vi "FP_Size Inside Bounds with Scrollbars.vi"(7 "WkSpace":T1, 8 "Error":errorcluster, 11 "VI":refnum<vi>) -> (0 "Error Out":errorcluster, 2 "Fit Successful":bool, 3 "VI Out":refnum<vi>)   [LabVIEW 2020]
uses:
  <vilib>/Utility/miscctls.llb/LVRectTypeDef.ctl
  TypeDefs_Utility/Cluster_FP_Scroll Bars Hide Show.ctl
  TypeDefs_Utility/ENUM_FP_Show-Hide Select.ctl
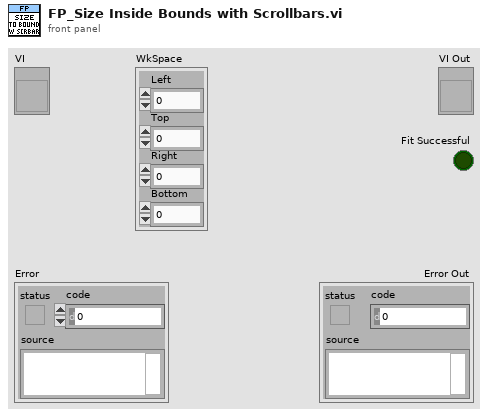
[diagram p1: front panel]
types:
  T1 = typedef "LVRectTypeDef.ctl" = cluster{"Left":i16, "Top":i16, "Right":i16, "Bottom":i16}
  T2 = typedef "Cluster_FP_Scroll Bars Hide Show.ctl" = cluster{"Horiz SBar":T3, "Vert SBar":T3}
  T3 = typedef "ENUM_FP_Show-Hide Select.ctl" = enum16{"No Change", "Hide", "Show"}
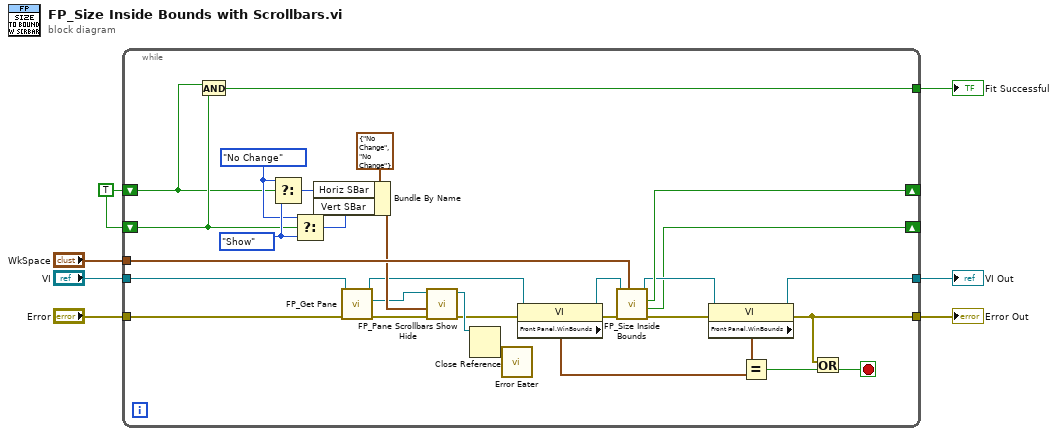
[diagram p0: block diagram]
diagram:
  w1 = TRUE ("Horizontal In Range Out")
  n1 = while {
    tunnel: [w14] -> w7
    tunnel: "VI" -> [w22]
    tunnel: "Error" -> [w21]
    tunnel: [w8] -> w4
    tunnel: [w37] -> w3
    tunnel: "WkSpace" -> [w36]
    shift-right: [w35] -> _
    shift-left: w1 -> [w23]
    shift-right: [w13] -> _
    shift-left: w1 -> [w24]
    stop <- w9 stop-if-true
    w26 = ENUM_FP_Show-Hide_Select."Show" ("Horizontal")
    w25 = ENUM_FP_Show-Hide_Select."No Change" ("Horizontal")
    n2 = And(x=w23, y=w24) -> (x .and. y?=w37:bool)
    n3 = Select(t=w25, s=w23, f=w26) -> (s? t:f=w31:T3)
    n4 = Select(t=w25, s=w24, f=w26) -> (s? t:f=w30:T3)
    n5 = Bundle By Name(cluster=T2 {"Horiz SBar"=enum."No Change", "Vert SBar"=enum."No Change"} ("Scrollbar Settings"), "Horiz SBar"=w31, "Vert SBar"=w30) -> (w32:T2)
    n6 = call "FP_Get Pane.vi"("Error"=w21, "VI"=w22) -> ("Error Out"=w27:errorcluster, "Pane Refnum Out"=w29:refnum<vi>, "VI Out"=w20:refnum<vi>)  [unwired: 7 in]
    n7 = call "FP_Pane Scrollbars Show Hide.vi"("Error"=w27, "Scrollbar Settings"=w32, "Pane"=w29) -> ("Error Out"=w18:errorcluster, "Pane Out"=w28:refnum<vi>)  [unwired: 7 in]
    n8 = Close Reference(reference=w28) -> (error out=w34:errorcluster)  [unwired: 1 in]
    n9 = call "Error Eater.vi"("error in (no error)"=w34) -> ()  [unwired: 2 in]
    n10 = property class="VI"(reference=w20, error in=w18) -> (reference out=w19:refnum<vi>, error out=w17:errorcluster, "Front Panel.WinBounds"=w11:T1)
    n11 = call "FP_Size Inside Bounds.vi"("Work Space"=w36, "Error"=w17, "VI Ref"=w19) -> ("Error Out"=w16:errorcluster, "Vertical In Range Out"=w13:bool, "Horizontal In Range Out"=w35:bool, "VI Ref Out"=w15:refnum<vi>)  [unwired: 3 in, 2 out]
    n12 = property class="VI"(reference=w15, error in=w16) -> (reference out=w14:refnum<vi>, error out=w8:errorcluster, "Front Panel.WinBounds"=w12:T1)
    n13 = Equal?(x=w12, y=w11) -> (x = y?=w10:bool)
    n14 = Or(x=w8, y=w10) -> (x .or. y?=w9:bool)
  }
  "VI Out" <- w7
  "Fit Successful" <- w3
  "Error Out" <- w4
